vi "GPIB interact.vi"() -> ()   [LabVIEW 2017]
panel:
  in  "address":string
  out "Writting error 2":errorcluster
  in  "command":string
  out "Reading error":errorcluster
  out "data":string
  in  "Inquiry?":bool
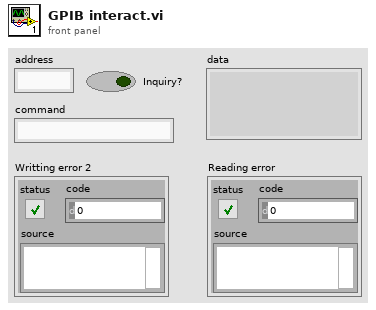
[diagram p1: front panel]
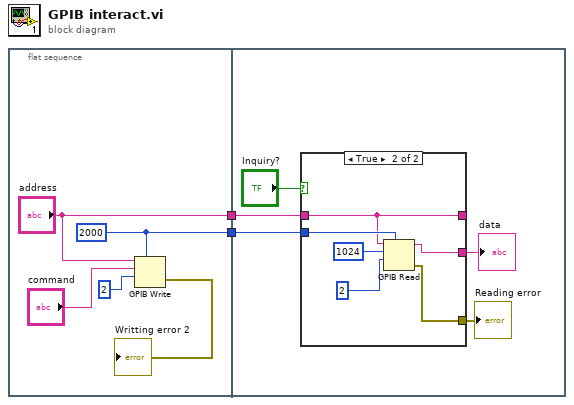
[diagram p0: block diagram]
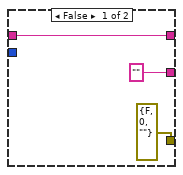
[diagram p2: hidden frame]
diagram:
  n1 = flat-sequence {
    tunnel: [w6] -> w2
    tunnel: ["address"] -> w1
    tunnel: w2 -> [w12]
    tunnel: w1 -> [w8]
    frame #0 {
      w6 = 2000 ("timeout ms (488.2 global)")
      n2 = GPIB Write(0:"address", 1:"command", 2:i16 2 ("mode (0)"), 4:w6) -> (6:→"Writting error 2":errorcluster)  [unwired: 1 in, 1 out]
    }
    frame #1 {
      n3 = case shown="True" "Inquiry?" {
        tunnel: ["" ("data") w20] -> w10
        tunnel: [errorcluster {"status"=FALSE, "code"=0, "source"=""} ("error out") w19] -> w11
        tunnel: w12 -> [_ w18]
        tunnel: w8 -> [w13 w16]
        tunnel: [w13 w16] -> _
        frame False {
        }
        frame True {
          n4 = GPIB Read(0:w16, 1:1024 ("byte count"), 2:i16 2 ("mode (0)"), 4:w18) -> (5:w20:string, 7:w19:errorcluster)  [unwired: 1 in, 1 out]
        }
      }
      "data" <- w10
      "Reading error" <- w11
    }
  }
